vi "Constructor.vi"(4 "TimeZoneInfoId":string, 5 "EndDate":timestamp, 6 "StepExecutionStatus":T1=enum."NOT_COMPLETED", 7 "StartDate":timestamp, 8 "error in":errorcluster, 10 "StepName":string, 11 "Name":string) -> (0 "error out":errorcluster, 3 "StepRun out":refnum<class "StepRun.lvclass">)   [LabVIEW 2021, in "ProligentXMLGenerator.lvlib" / "StepRun.lvclass"]
uses:
  StepRun.lvclass
  StepRun.lvclass/StepRun.ctl
  Base/DateTime/DateTime.lvclass
  Base/ExecutionStatus/ExecutionStatus.lvclass
  Measure/Measure/Measure.lvclass
  Base/NonEmptyString_255/NonEmptyString_255.lvclass
  Data.ctl
  Base/Guid/Guid.lvclass
  Model/CustomData/CustomData.lvclass
  Model/Document/Document.lvclass
  Model/Characteristic/Characteristic.lvclass
  Failure/FailureReference/FailureReference.lvclass
  Base/ExecutionStatus/Value.ctl
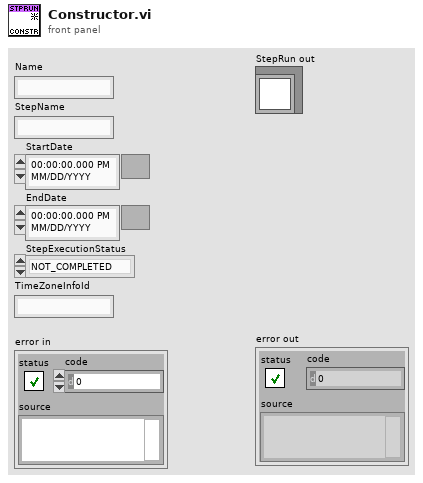
[diagram p1: front panel]
types:
  T1 = typedef "ProligentXMLGenerator.lvlib/ExecutionStatus.lvclass/Value.ctl" = enum16{"PASS", "FAIL", "NOT_COMPLETED", "ABORTED"}
  T2 = typedef "ProligentXMLGenerator.lvlib/StepRun.lvclass/Data.ctl" = cluster{"Name":string, "Measures":refnum<class "Measure.lvclass">[], "FailureReferences":refnum<class "FailureReference.lvclass">[], "Characteristics":refnum<class "Characteristic.lvclass">[], "Documents":refnum<class "Document.lvclass">[], "CustomData":refnum<class "CustomData.lvclass">, "StepExecutionStatus":refnum<class "ExecutionStatus.lvclass">, "StepRunId":refnum<class "Guid.lvclass">, "StepName":refnum<class "NonEmptyString_255.lvclass">, "StartDate":refnum<class "DateTime.lvclass">, "EndDate":refnum<class "DateTime.lvclass">, "TimeZoneInfoId":string}
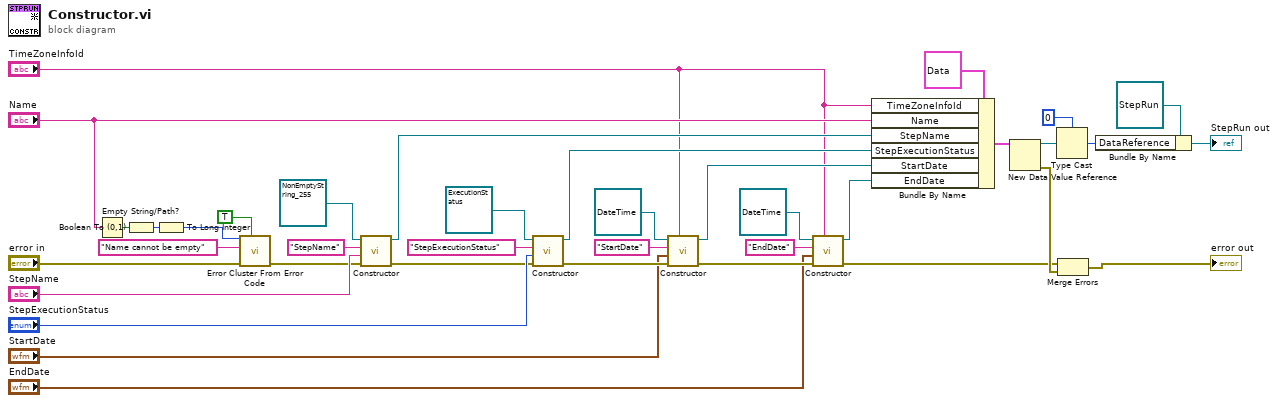
[diagram p0: block diagram]
diagram:
  n1 = Empty String/Path?(string/path="Name") -> (empty?=w23:bool)
  n2 = Boolean To (0,1)(Boolean=w23) -> (0, 1=w22:i16)
  n3 = To Long Integer(number=w22) -> (32bit integer=w21:i32)
  n4 = call <vilib>:"Error Cluster From Error Code.vi"("show call chain? (False)"=TRUE, "error in (no error)"="error in", "error message (\"\")"="Name cannot be empty" ("error message (\"\")"), "error code (0)"=w21) -> ("error out"=w19:errorcluster)  [unwired: 5 in]
  n5 = call-dynamic "Constructor.vi"("error in"=w19, "Value"="StepName", "Name"="StepName", "String in"=refnum<class "NonEmptyString_255.lvclass"> refnum ("ProligentResultProcessor:NonEmptyString_255")) -> ("error out"=w12:errorcluster, "String out"=w17:refnum<class "NonEmptyString_255.lvclass">)  [unwired: 6 in]
  n6 = call-dynamic "Constructor.vi"("error in"=w12, "Value"="StepExecutionStatus", "Name"="StepExecutionStatus", "ExecutionStatus in"=refnum<class "ExecutionStatus.lvclass"> refnum ("ProligentResultProcessor:ExecutionStatus")) -> ("error out"=w16:errorcluster, "ExecutionStatus out"=w13:refnum<class "ExecutionStatus.lvclass">)  [unwired: 6 in]
  n7 = call-dynamic "Constructor.vi"("TimeZoneInfoId"="TimeZoneInfoId", "error in"=w16, "Value"="StartDate", "Name"="StartDate", "DateTime in"=refnum<class "DateTime.lvclass"> refnum) -> ("error out"=w7:errorcluster, "DateTime out"=w25:refnum<class "DateTime.lvclass">)  [unwired: 5 in]
  n8 = call-dynamic "Constructor.vi"("TimeZoneInfoId"="TimeZoneInfoId", "error in"=w7, "Value"="EndDate", "Name"="EndDate", "DateTime in"=refnum<class "DateTime.lvclass"> refnum) -> ("error out"=w6:errorcluster, "DateTime out"=w5:refnum<class "DateTime.lvclass">)  [unwired: 5 in]
  n9 = Bundle By Name(cluster=T2 {"Name"="", "Measures"=[], "FailureReferences"=[], "Characteristics"=[], "Documents"=[], "CustomData"=refnum, "StepExecutionStatus"=refnum, "StepRunId"=refnum, "StepName"=refnum, "StartDate"=refnum, "EndDate"=refnum, "TimeZoneInfoId"=""} ("Data"), "TimeZoneInfoId"="TimeZoneInfoId", "Name"="Name", "StepName"=w17, "StepExecutionStatus"=w13, "StartDate"=w25, "EndDate"=w5) -> (w30:T2)
  n10 = New Data Value Reference(data value=w30) -> (data value reference=w29:refnum<data-value>, error out=w26:errorcluster)  [unwired: 1 in]
  n11 = Type Cast(type=u64 0, x=w29) -> (*(type *) &x=w27:u64)
  n12 = Merge Errors(w6, w26) -> (→"error out":errorcluster)
  n13 = Bundle By Name(cluster=refnum<class "StepRun.lvclass"> refnum ("ProligentResultProcessor:StepRun"), "DataReference"=w27) -> (→"StepRun out":refnum<class "StepRun.lvclass">)
